vi "Write Config.lvclass.vi"(8 "error in (no error)":errorcluster, 10 "Config.lvclass":refnum<class "Config.lvclass">, 11 "DelayLine in":refnum<class "DelayLine.lvclass">) -> (0 "error out":errorcluster, 3 "DelayLine out":refnum<class "DelayLine.lvclass">)   [LabVIEW 2015]
uses:
  dependecies/ControlsVIs/Clusters-def/SERVER-Commands.ctl
  DelayLine.lvclass
  Config/Config.lvclass
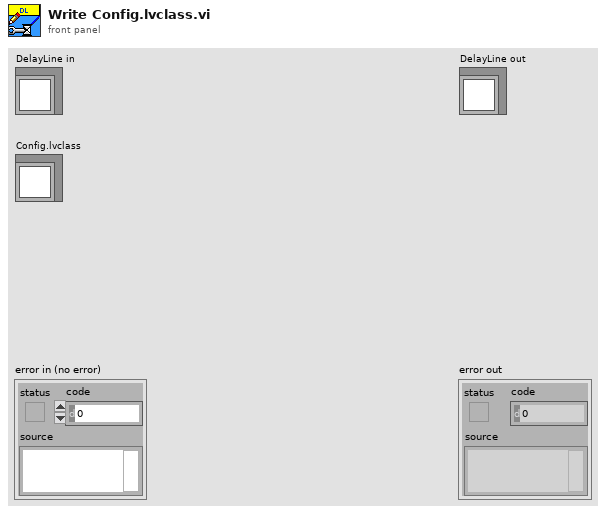
[diagram p1: front panel]
types:
  T1 = typedef "SERVER-Commands.ctl" = string
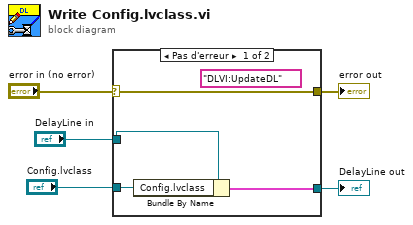
[diagram p0: block diagram]
diagram:
  n1 = case shown="Pas d'erreur" "error in (no error)" {
    selector: "error in (no error)" -> [w6 w10]
    tunnel: [w6 w10] -> w4
    tunnel: [w7 w11] -> w2
    tunnel: "DelayLine in" -> [w8 w11]
    tunnel: "Config.lvclass" -> [w9 _]
    frame No Error {
      (unwired) T1 "DLVI:UpdateDL" ("Commands")
      n2 = Bundle By Name(cluster=w8, "Config.lvclass"=w9) -> (w7:cluster{})
    }
    frame Error {
    }
  }
  "error out" <- w4
  "DelayLine out" <- w2
